vi "Test_Zip.vi"() -> (0 "error out":errorcluster, 8 "File to transfer":path[](array[path]))   [LabVIEW 2012]
panel:
  in  "Folder to Zip":path
  in  "Folder to create Zip File in":path
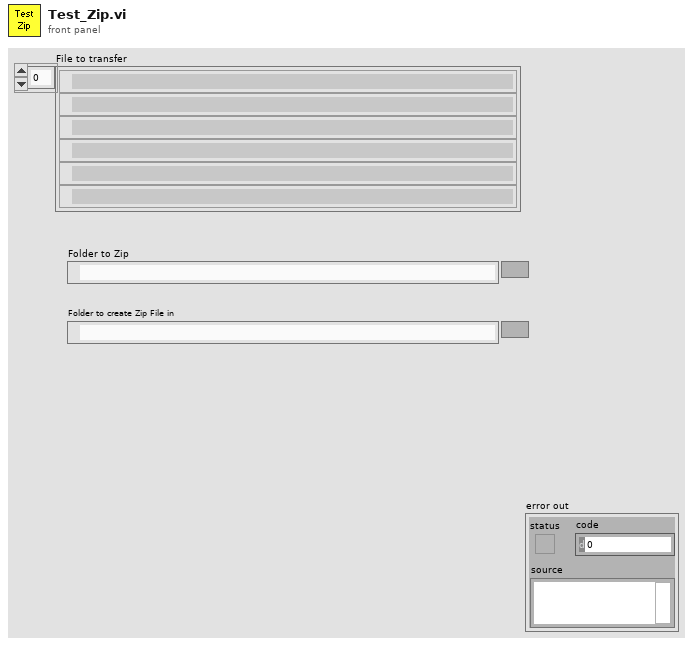
[diagram p1: front panel]
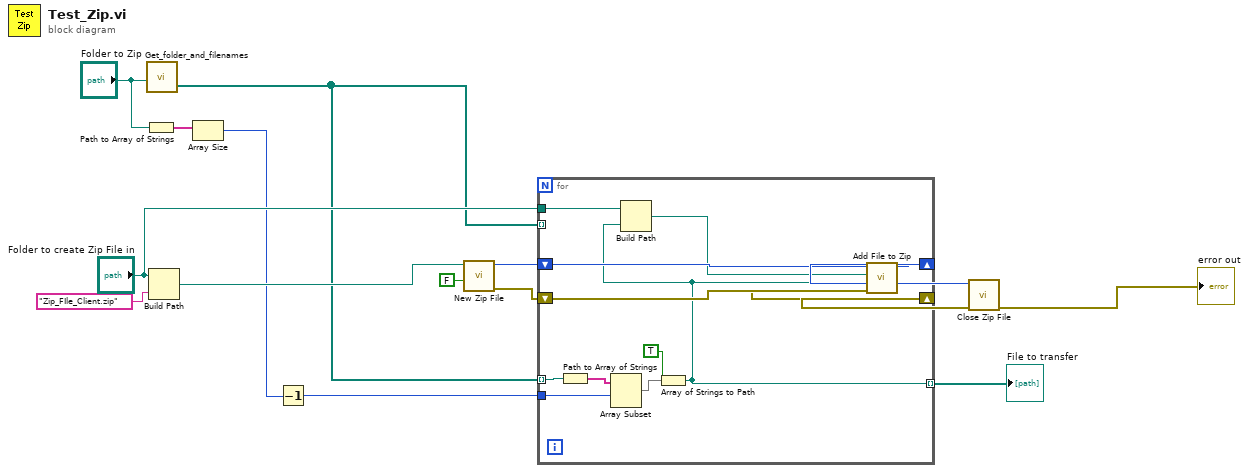
[diagram p0: block diagram]
diagram:
  n1 = Path to Array of Strings(0:"Folder to Zip") -> (2:w4:string[])  [unwired: 1 out]
  n2 = call "Get_folder_and_filenames.vi"("file path (dialog if empty)"="Folder to Zip") -> ("Files"=w5:path[])  [unwired: 1 out]
  n3 = Build Path(base path="Folder to create Zip File in", name or relative path="Zip_FIle_Client.zip") -> (appended path=w14:path)
  n4 = Array Size(array=w4) -> (size(s)=w3:i32)
  n5 = Decrement(x=w3) -> (x-1=w1:i32)
  n6 = call <vilib>:"New Zip File.vi"("confirm overwrite? (F)"=FALSE, "target"=w14) -> ("error out"=w10:errorcluster, "zip file out"=w12:i64)  [unwired: 3 in, 1 out]
  n7 = for {
    shift-right: [w26] -> w13
    shift-left: w12 -> [w27]
    tunnel: "Folder to create Zip File in" -> [w25]
    tunnel: w5 -> [_] mode=indexing
    shift-right: [w22] -> w9
    shift-left: w10 -> [w23]
    tunnel: w5 -> [w21] mode=indexing
    tunnel: w1 -> [w18]
    tunnel: [w17] -> w2 mode=indexing
    n8 = Path to Array of Strings(0:w21) -> (2:w20:string[])  [unwired: 1 out]
    n9 = Array Subset(array=w20, index=w18) -> (w19:string[])  [unwired: 1 in]
    n10 = Array of Strings to Path(0:w19, 1:TRUE ("relative")) -> (2:w17:path)
    n11 = Build Path(base path=w25, name or relative path=w17) -> (appended path=w24:path)
    n12 = call <vilib>:"Add File to Zip.vi"("error in (no error)"=w23, "destination path in zip"=w17, "source file path"=w24, "zip file in"=w27) -> ("error out"=w22:errorcluster, "zip file out"=w26:i64)  [unwired: 6 in]
  }
  "File to transfer" <- w2
  n13 = call <vilib>:"Close Zip File.vi"("error in (no error)"=w9, "zip file in"=w13) -> ("error out"=→"error out":errorcluster)  [unwired: 5 in]
